vi "Async.Engine.Close.vi"(8 "error in":errorcluster, 11 "VS Plugin Inline Async API in":refnum<class "VS Plugin Inline Async API.lvclass">) -> (0 "error out":errorcluster, 3 "VS Plugin Inline Async API out":refnum<class "VS Plugin Inline Async API.lvclass">)   [LabVIEW 2024, in "VS Plugin Inline Async API.lvlib" / "VS Plugin Inline Async API.lvclass"]
uses:
  VS Plugin Inline Async API.lvclass
  VS Plugin Inline Async API.lvclass/VS Plugin Inline Async API.ctl
  Plugin Data Access Engine/Data Access Engine/Plugin Data Access Engine.lvclass
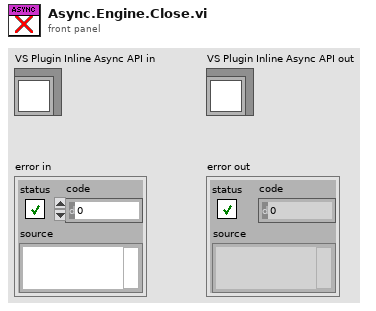
[diagram p1: front panel]
types:
  T1 = typedef "VS Plugin Inline Async API.lvlib/VS Plugin Inline Async API.lvclass/Error Handling Settings.ctl" = cluster{"Write to SystemLog (F)":bool}
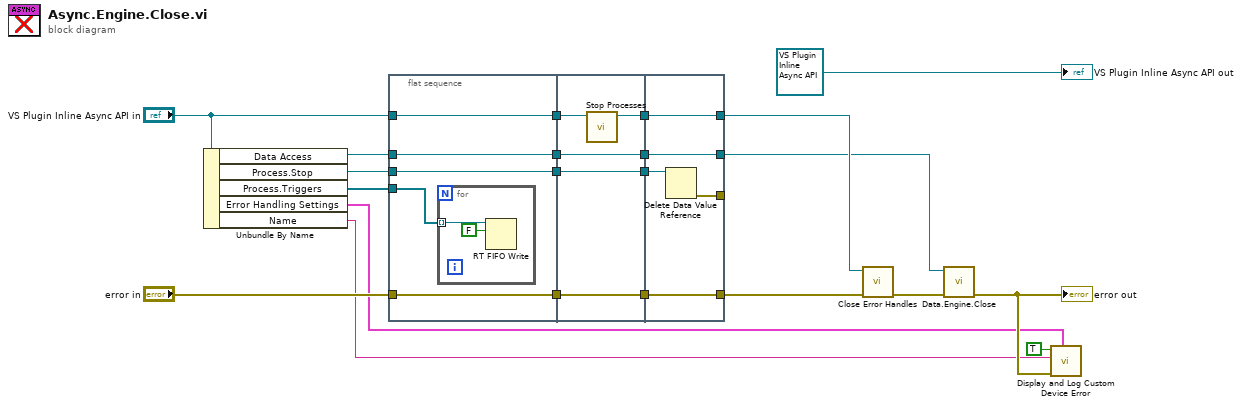
[diagram p0: block diagram]
diagram:
  n1 = Unbundle By Name("VS Plugin Inline Async API in") -> ("Data Access"=w4:refnum<class "Plugin Data Access Engine.lvclass">, "Process.Stop"=w7:refnum<data-value>, "Process.Triggers"=w3:refnum<k33>[], "Error Handling Settings"=w2:T1, "Name"=w8:string)
  n2 = flat-sequence {
    tunnel: [w27] -> w22
    tunnel: "error in" -> [w27]
    tunnel: [w26] -> w15
    tunnel: "VS Plugin Inline Async API in" -> [w26]
    tunnel: w7 -> [w25]
    tunnel: [w25] -> w14
    tunnel: [w24] -> w13
    tunnel: w4 -> [w24]
    tunnel: w3 -> [w23]
    tunnel: [w34] -> w21
    tunnel: w22 -> [w34]
    tunnel: w15 -> [w31]
    tunnel: [w33] -> w12
    tunnel: w14 -> [w33]
    tunnel: [w30] -> w11
    tunnel: [w32] -> w10
    tunnel: w13 -> [w32]
    tunnel: [w39] -> w20
    tunnel: w21 -> [w39]
    tunnel: w12 -> [w37]
    tunnel: [w36] -> w6
    tunnel: w11 -> [w36]
    tunnel: [w38] -> _
    tunnel: [w35] -> w5
    tunnel: w10 -> [w35]
    frame #0 {
      n3 = for {
        tunnel: w23 -> [w29] mode=indexing
        n4 = RT FIFO Write(0:w29, 1:FALSE ("element")) -> ()  [unwired: 3 in, 4 out]
      }
    }
    frame #1 {
      n5 = call "Stop Processes.vi"("VS Plugin Inline Async API in"=w31) -> ("VS Plugin Inline Async API out"=w30:refnum<class "VS Plugin Inline Async API.lvclass">)  [unwired: 10 in]
    }
    frame #2 {
      n6 = Delete Data Value Reference(data value reference=w37) -> (error out=w38:errorcluster)  [unwired: 1 in, 1 out]
    }
  }
  n7 = call "Close Error Handles.vi"("error in"=w20, "VS Plugin Inline Async API in"=w6) -> ("error out"=w19:errorcluster)  [unwired: 8 in, 1 out]
  n8 = call "Data.Engine.Close.vi"("error in"=w19, "Plugin Data Access in"=w5) -> ("error out"=w18:errorcluster)  [unwired: 8 in, 1 out]
  "error out" <- w18
  n9 = call "Display and Log Custom Device Error.vi"("Error Log Settings"=w2, "error out"=w18, "Your code's public name"=w8, "Custom Device? (T)"=TRUE) -> ()  [unwired: 8 in]
  "VS Plugin Inline Async API out" <- refnum<class "VS Plugin Inline Async API.lvclass"> refnum ("VS Plugin Inline Async API out")
